vi "HW operation.vi"(1 "operation2":dbl, 2 "operation":string(combo), 3 "operation1":dbl) -> (0 "results":dbl)   [LabVIEW 2018]
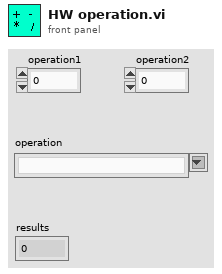
[diagram p1: front panel]
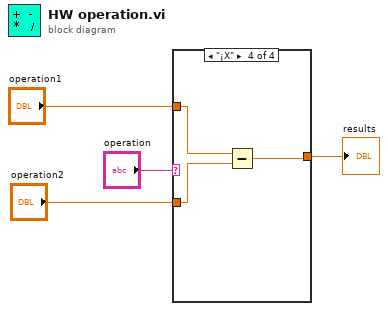
[diagram p0: block diagram]
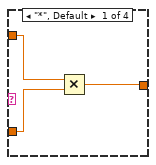
[diagram p2: hidden frame]
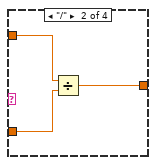
[diagram p3: hidden frame]
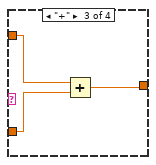
[diagram p4: hidden frame]
diagram:
  n1 = case shown="\"¡X\"" "operation" {
    tunnel: "operation1" -> [w6 w10 w12 w15]
    tunnel: "operation2" -> [w5 w9 w11 w14]
    tunnel: [w7 w8 w13 w16] -> w1
    frame "*", Default {
      n2 = Multiply(x=w6, y=w5) -> (x*y=w7:dbl)
    }
    frame "/" {
      n3 = Divide(x=w10, y=w9) -> (x/y=w8:dbl)
    }
    frame "+" {
      n4 = Add(x=w12, y=w11) -> (x+y=w13:dbl)
    }
    frame "¡X" {
      n5 = Subtract(x=w15, y=w14) -> (x-y=w16:dbl)
    }
  }
  "results" <- w1
